vi "Calibration Get Channels DAQ Parameters From SencorConfig Table.vi"(8 "error in (no error)":errorcluster, 11 "Main":string) -> (0 "error out":errorcluster, 2 "Single Channel DAQ Parameters":T1, 3 "DAQ Parameters":T1[](array[typedef]))   [LabVIEW 2017, in "SQLite.lvclass"]
doc: "in put the sensors name list \nget each channel MuliplyFactor ,RawPrecision, PhysicalPrecision"
uses:
  SQLite.lvclass
  DAQParameters.ctl
  <userlib>/sushu/sushu.lvlib
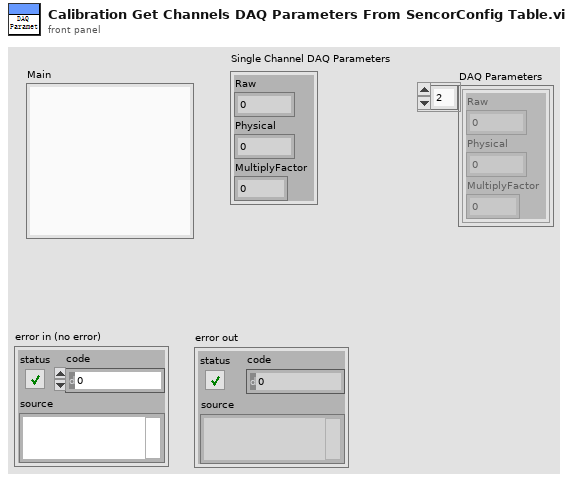
[diagram p1: front panel]
types:
  T1 = typedef "SQLite.lvclass/DAQParameters.ctl" = cluster{"Raw":i16, "Physical":i16, "MultiplyFactor":dbl}
  T2 = enum16{"SelectAllData", "SelectDataBySensorName"}
  T3 = cluster{"[0]":T1, "[1]":T1, "[2]":T1, "[3]":T1, "[4]":T1, "[5]":T1, "[6]":T1, "[7]":T1, "[8]":T1, "[9]":T1, "[10]":T1, "[11]":T1, "[12]":T1, "[13]":T1, "[14]":T1}
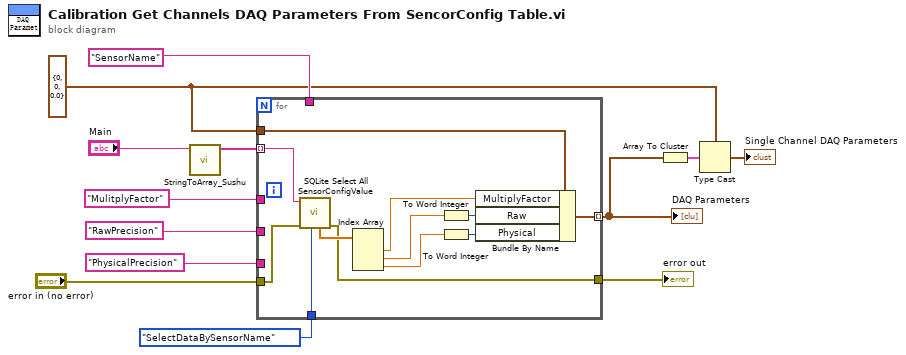
[diagram p0: block diagram]
diagram:
  w4 = T1 {"Raw"=0, "Physical"=0, "MultiplyFactor"=0.0} ("DAQParameters")
  n1 = call <userlib>:"StringToArray_Sushu.vi"("State Queue"="Main") -> ("Array"=w12:string[])  [unwired: 8 in, 2 out]
  n2 = for {
    tunnel: "SensorName" ("Main") -> [_]
    tunnel: "PhysicalPrecision" ("VariableName") -> [_]
    tunnel: "RawPrecision" ("VariableName") -> [_]
    tunnel: "MulitplyFactor" ("VariableName") -> [_]
    tunnel: [w23] -> w5 mode=indexing
    tunnel: w4 -> [w22]
    tunnel: "error in (no error)" -> [w15]
    tunnel: w12 -> [w21] mode=indexing
    tunnel: T2."SelectDataBySensorName" ("ALL/Single") -> [w20]
    tunnel: [w14] -> w1
    n3 = call "SQLite Select All SensorConfigValue.vi"("ALL/Single"=w20, "error in (no error)"=w15, "SensorName"=w21) -> ("error out"=w14:errorcluster, "Factor/SensorPrecision/ChannelPrecision"=w19:dbl[])  [unwired: 3 in, 4 out]
    n4 = Index Array(array=w19) -> (element #1=w18:dbl, element #2=w17:dbl, element #3=w16:dbl)  [unwired: 3 in]
    n5 = To Word Integer(number=w17) -> (16bit integer=w25:i16)
    n6 = To Word Integer(number=w16) -> (16bit integer=w24:i16)
    n7 = Bundle By Name(cluster=w22, "MultiplyFactor"=w18, "Raw"=w25, "Physical"=w24) -> (w23:T1)
  }
  "error out" <- w1
  "DAQ Parameters" <- w5
  n8 = Array To Cluster(array=w5) -> (cluster=w6:T3)
  n9 = Type Cast(type=w4, x=w6) -> (*(type *) &x=→"Single Channel DAQ Parameters":T1)
